vi "Generator_a.vi"(0 "Stop":bool caption="Start/Stop") -> (4 "Generated_Data":dbl caption="Generated Data")   [LabVIEW 2021]
doc: "This VI continuously generate Data and push it to the Acquisition VI.\nTransfer of thet data happens under Global variable."
uses:
  Global_Variables/Generate_Data_Global.vi
  <vilib>/numeric/Random Number (Range) DBL.vi
panel:
  in  "Error_In":errorcluster
  out "Error_Out":errorcluster
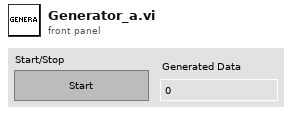
[diagram p1: front panel]
types:
  T1 = enum16{"Left Button", "Center Button", "Right Button", "Window Close"}
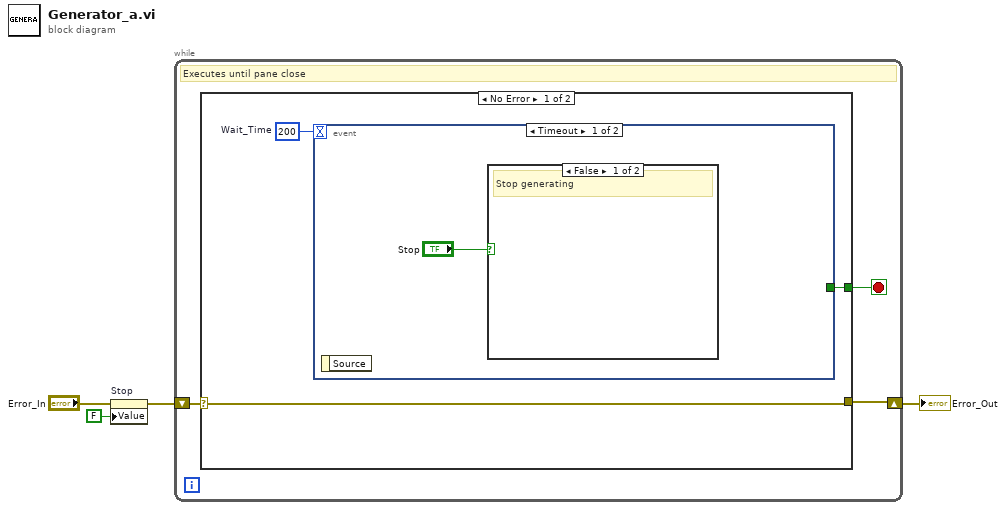
[diagram p0: block diagram]
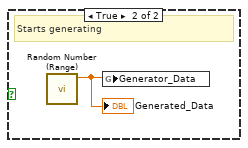
[diagram p2: hidden frame]
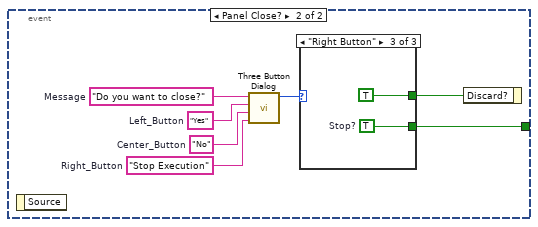
[diagram p3: hidden frame]
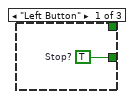
[diagram p4: hidden frame]
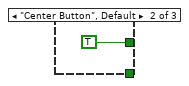
[diagram p5: hidden frame]
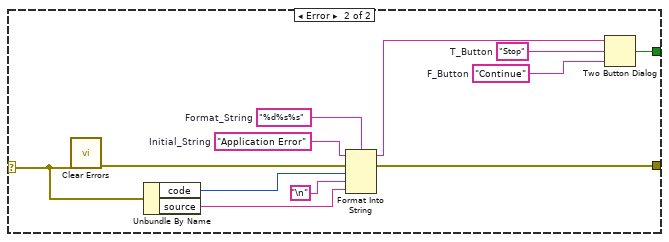
[diagram p6: hidden frame]
diagram:
  n1 = property on="Stop" class="Bool (strict)"(error in="Error_In", "Value"=FALSE ("Stop")) -> (error out=w2:errorcluster)  [unwired: 1 in, 1 out]
  n2 = while {
    shift-right: [w6] -> w4
    shift-left: w2 -> [w5]
    stop <- w7 stop-if-true
    # "Executes until pane close"
    n3 = case shown="No Error" w5 {
      selector: w5 -> [w8 w26]
      tunnel: [w9 w24] -> w7
      tunnel: [w8 w25] -> w6
      frame No Error {
        w10 = 200  # Wait_Time
        n4 = event shown="[0] Timeout" {
          selector: _ -> [_ _]
          dyn-events: _ -> [_ _]
          timeout: w10 -> [_ _]
          tunnel: [_ w13] -> w9
          event Timeout {
            n5 = event-data() -> ()  [unwired: 1 in, 1 out]
            n6 = case shown="False" "Stop" {
              frame False {
                # "Stop generating"
              }
              frame True {
                # "Starts generating"
                n7 = call-poly <vilib>:"Random Number (Range).vi"() -> ("number"=w12:dbl)  [unwired: 11 in]
                "Generated_Data" <- w12
                n8 = global write "Generate_Data_Global.vi" "Generator_Data"(w12) -> ()
              }
            }
          }
          event Panel Close? {
            w16 = "Stop Execution"  # Right_Button
            w17 = "No"  # Center_Button
            w18 = "Yes"  # Left_Button
            w19 = "Do you want to close?"  # Message
            n9 = event-data() -> ()  [unwired: 1 in, 1 out]
            n10 = call <vilib>:"Three Button Dialog.vi"("Right Button Text (\"Cancel\")"=w16, "Center Button Text (\"No\")"=w17, "Left Button Text (\"Yes\")"=w18, "message"=w19) -> ("Which Button?"=w15:T1)  [unwired: 7 in]
            n11 = case shown="\"Right Button\"" w15 {
              tunnel: [_ TRUE ("Discard?") TRUE ("Discard?")] -> w14
              tunnel: [w20 _ w23] -> w13
              frame "Left Button" {
                w20 = TRUE  # Stop?
              }
              frame "Center Button", Default {
              }
              frame "Right Button" {
                w23 = TRUE  # Stop?
              }
            }
            n12 = event-data("Discard?"=w14) -> ()  [unwired: 1 in, 1 out]
          }
        }
      }
      frame Error {
        w31 = "%d%s%s"  # Format_String
        w32 = "Application Error"  # Initial_String
        w33 = "Stop"  # T_Button
        w34 = "Continue"  # F_Button
        n13 = call <vilib>:"Clear Errors.vi"("error in (no error)"=w26) -> ("error out"=w29:errorcluster)  [unwired: 5 in, 1 out]
        n14 = Unbundle By Name(w26) -> ("code"=w28:i32, "source"=w27:string)
        n15 = Format Into String(format string=w31, initial string=w32, error in=w29, w28, "\n", w27) -> (resulting string=w35:string, error out=w25:errorcluster)
        n16 = Two Button Dialog(message=w35, 1:w34, 2:w33) -> (T button?=w24:bool)
      }
    }
  }
  "Error_Out" <- w4
